vi "AddOccurrence.vi"(7 "nonEmpty":bool, 8 "occ":refnum<k4>, 11 "SubChannel in":refnum<class "SubChannelCPU.lvclass">) -> (3 "SubChannel out":refnum<class "SubChannelCPU.lvclass">)   [LabVIEW 2019, in "MessengerM.lvlib" / "SubChannelCPU.lvclass"]
uses:
  SubChannelCPU.lvclass
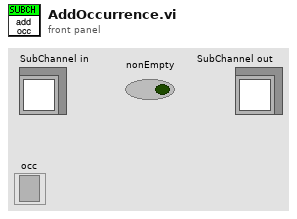
[diagram p1: front panel]
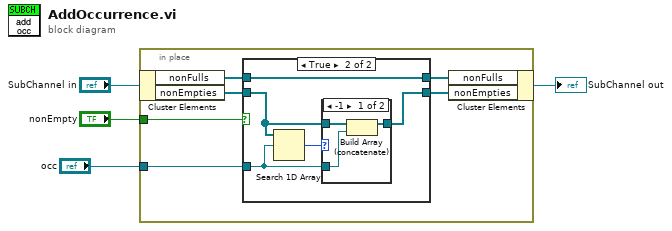
[diagram p0: block diagram]
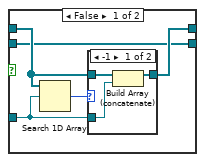
[diagram p2: hidden frame]
diagram:
  n1 = in-place {
    in-place-border: "nonEmpty" -> [w10]
    in-place-border: "occ" -> [w5]
    n2 = in-place-cluster #1("SubChannel in") -> ("nonFulls"=w7:refnum<k4>[], "nonEmpties"=w9:refnum<k4>[])
    n3 = case shown="True" w10 {
      tunnel: w9 -> [w11 w22]
      tunnel: [w13 w20] -> w8
      tunnel: w7 -> [w12 w20]
      tunnel: [w11 w21] -> w6
      tunnel: w5 -> [w14 w23]
      frame False {
        n4 = Search 1D Array(1D array=w12, element=w14) -> (index of element=w15:i32)  [unwired: 1 in]
        n5 = case shown="-1" w15 {
          tunnel: w12 -> [w18 w19]
          tunnel: w14 -> [w17 _]
          tunnel: [w16 w19] -> w13
          frame -1 {
            n6 = Build Array (concatenate)(w18, w17) -> (w16:refnum<k4>[])
          }
          frame Default {
          }
        }
      }
      frame True {
        n7 = Search 1D Array(1D array=w22, element=w23) -> (index of element=w24:i32)  [unwired: 1 in]
        n8 = case shown="-1" w24 {
          tunnel: w22 -> [w27 w28]
          tunnel: w23 -> [w26 _]
          tunnel: [w25 w28] -> w21
          frame -1 {
            n9 = Build Array (concatenate)(w27, w26) -> (w25:refnum<k4>[])
          }
          frame Default {
          }
        }
      }
    }
    n10 = in-place-cluster #1("nonFulls"=w8, "nonEmpties"=w6) -> (→"SubChannel out":refnum<class "SubChannelCPU.lvclass">)
  }
